vi "Serial_Configuration.vi"(0 "VISA resource name":refnum<visa-resource-name>, 1 "baud rate (9600)":u32=9600, 2 "data bits (8)":u16=8 min=5 max=8 step=1, 3 "parity (0:none)":enum16{"None", "Odd", "Even", "Mark", "Space"}(ring), 5 "error in (no error)":errorcluster, 6 "timeout (10sec)":u32=10000, 8 "termination char\n(0xA = '\\n' = LF)":u8=10 format="%.0x", 9 "stop bits (10: 1 bit)":u16(ring)=10 items=["1.0"=10, "1.5"=15, "2.0"=20], 10 "Enable Termination\nChar (T)":bool=TRUE, 11 "flow control (0:none)":u16(ring) items=["None", "XON/XOFF", "RTS/CTS", "XON/XOFF & RTS/CTS", "DTR/DSR", "XON/XOFF & DTR/DSR"]) -> (14 "VISA resource name out":refnum<visa-resource-name>, 16 "Chosen com is opened!":bool, 19 "error out":errorcluster)   [LabVIEW 2020]
uses:
  <vilib>/Instr/_visa.llb/VISA Configure Serial Port (Instr).vi
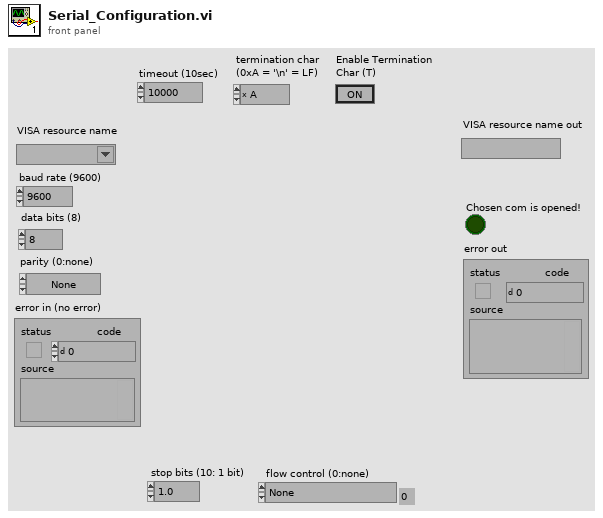
[diagram p1: front panel]
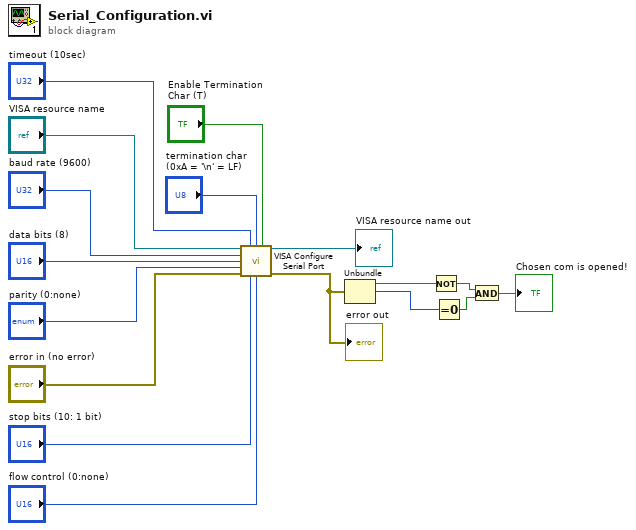
[diagram p0: block diagram]
diagram:
  n1 = call-poly "VISA Configure Serial Port"("VISA resource name"="VISA resource name", "timeout (10sec)"="timeout (10sec)", "termination char\n(0xA = '\\n' = LF)"="termination char\n(0xA = '\\n' = LF)", "Enable Termination\nChar (T)"="Enable Termination\nChar (T)", "baud rate (9600)"="baud rate (9600)", "data bits (8)"="data bits (8)", "parity (0:none)"="parity (0:none)", "error in (no error)"="error in (no error)", "stop bits (10: 1 bit)"="stop bits (10: 1 bit)", "flow control (0:none)"="flow control (0:none)") -> ("VISA resource name out"=→"VISA resource name out":refnum<visa-resource-name>, "error out"=w15:errorcluster)  [unwired: 4 in]
  "error out" <- w15
  n2 = Unbundle(w15) -> ("status"=w5:bool, "code"=w4:i32)  [unwired: 1 out]
  n3 = Not(x=w5) -> (.not. x?=w2:bool)
  n4 = Equal To 0?(x=w4) -> (x = 0?=w3:bool)
  n5 = And(x=w2, y=w3) -> (x .and. y?=→"Chosen com is opened!":bool)
